vi "server.vi"() -> ()   [LabVIEW 2020]
uses:
  System.Windows.Forms
  TCP Multiple Connections Data.ctl
  <userlib>/_MGI/Menu Building/MenuTypes/MenuStrip/MGI_MenuStrip.lvclass
  <userlib>/_MGI/Menu Building/MenuItemStatusChange/MGI_MenuItemStatusChange.lvclass
panel:
  in  "计划产量":u16 format="%d 件"
  in  "产品型号":u16(ring) items=[""=0, "R128"=1, "R527"=4, "R538"=5, "R92A"=3]
  out "完成率":sgl format="%_3f %"
  out "剩余数量":u16 format="%d 件"
  out "生产数量":u16 format="%d 件"
  out "布尔":bool
  out "停止":bool
  in  "菜单":refnum<k24>(container)
  in  "标题":string="Andon看板"
  out "备份4":T1(xcontrol)
  out "备份3":T1(xcontrol)
  out "备份2":T1(xcontrol)
  out "上转向轴总成、\n上柱管分总成拉拔力检测机":T1(xcontrol)
  out "GP12":T1(xcontrol)
  out "激光检测机":T1(xcontrol)
  out "最终功能测试+NVH 2":T1(xcontrol)
  out "最终功能测试+NVH 1":T1(xcontrol)
  out "传感器检测标定":T1(xcontrol)
  out "调节机构检测":T1(xcontrol)
  out "调节机构螺母拧紧\n扭矩检测机":T1(xcontrol)
  out "上柱管总成装配、\n滑移力检测":T1(xcontrol)
  out "中间轴装配":T1(xcontrol)
  out "控制器支架及电机装配":T1(xcontrol)
  out "上转向轴滑移力检测机":T1(xcontrol)
  out "上转向轴组件压装力检测机":T1(xcontrol)
  out "上/下柱管分总成压装力\n及拧紧扭矩检测机":T1(xcontrol)
  out "上柱管组件压装力检测机":T1(xcontrol)
  out "减速机构NVH测试评价":T1(xcontrol)
  out "双工位磨合试验机":T1(xcontrol)
  out "在线设备":i32 format="%.0d 台"
  # "芜湖恒隆汽车转向系统有限公司"
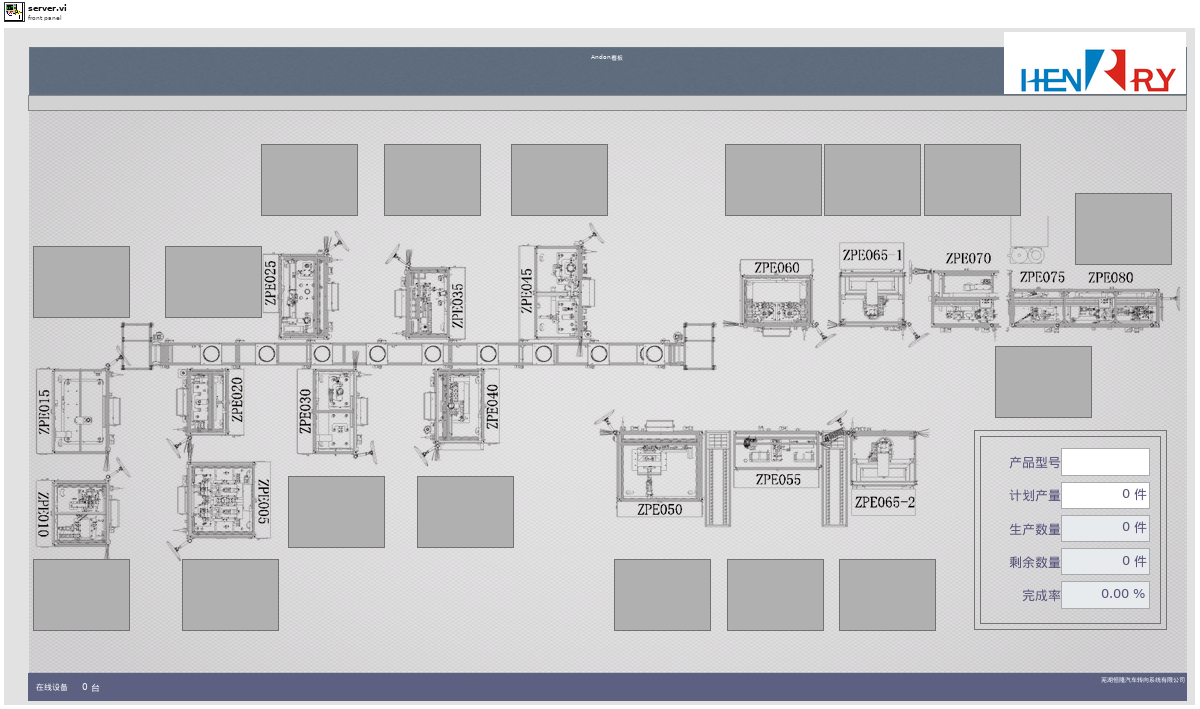
[diagram p1: front panel]
types:
  T1 = cluster{"设备名称":string, "操作人员":string, "设备状态":enum16{"设备离线", "设备正常", "设备缺料", "设备故障", "质量报警"}, "附加信息":string}
  T2 = typedef "TCP Multiple Connections Data.ctl" = cluster{"客户端":refnum<k5>[], "侦听器":refnum<k5>, "上线设备":string[]}
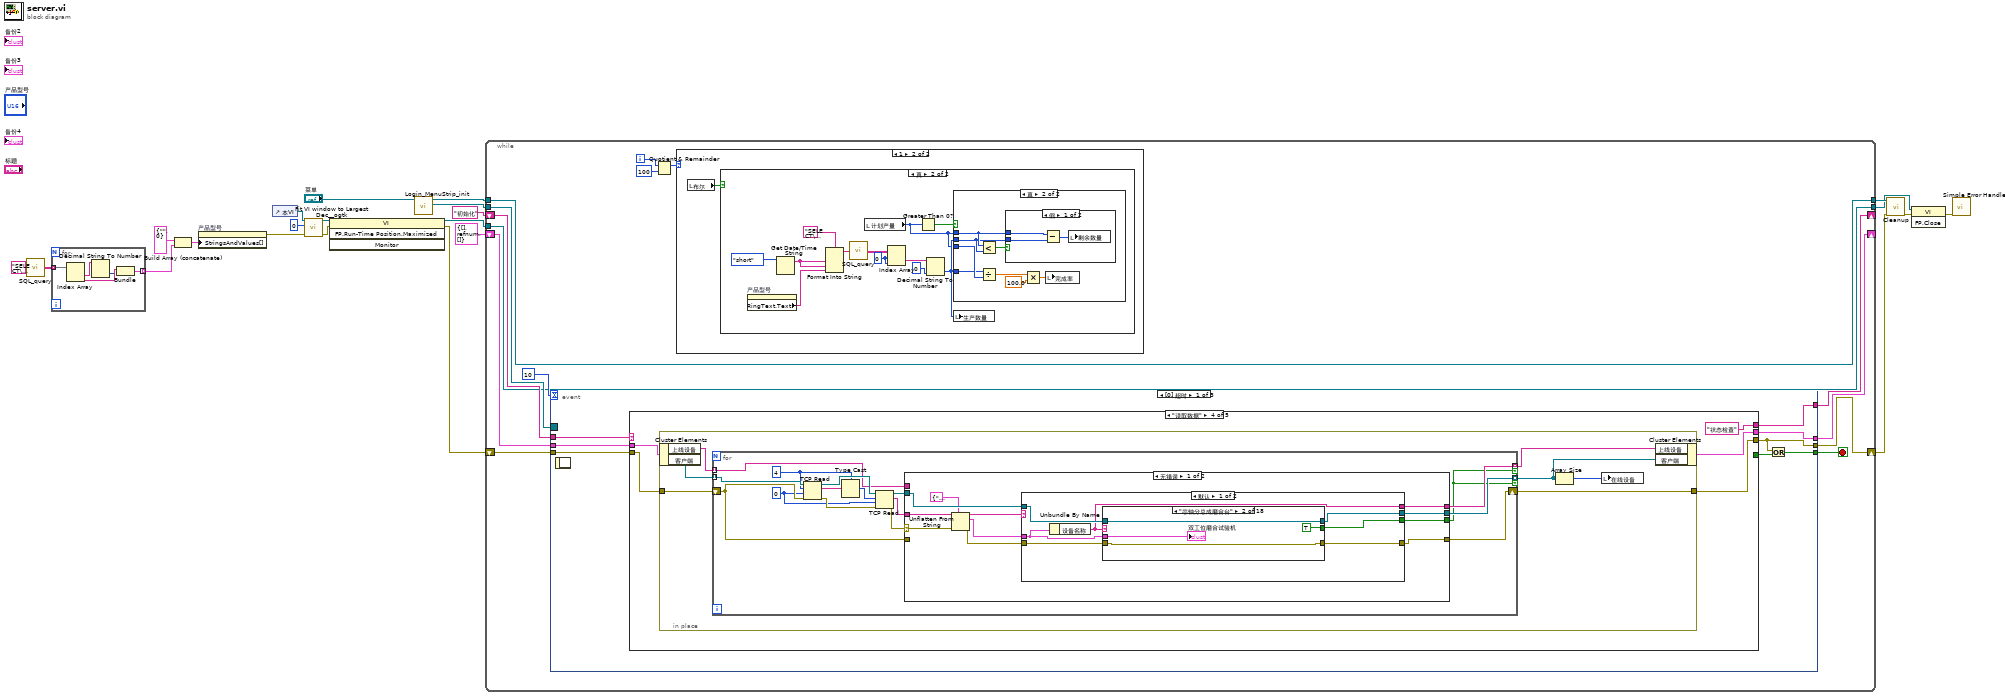
[diagram p0: block diagram]
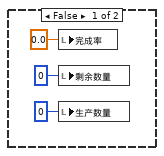
[diagram p3: hidden frame]
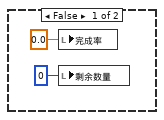
[diagram p4: hidden frame]
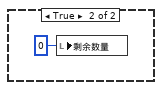
[diagram p5: hidden frame]
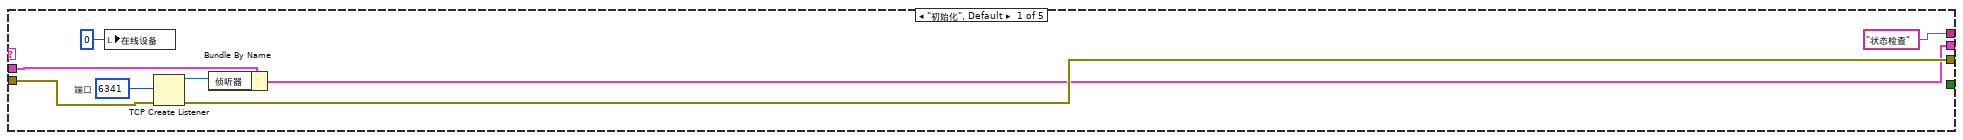
[diagram p6: hidden frame]
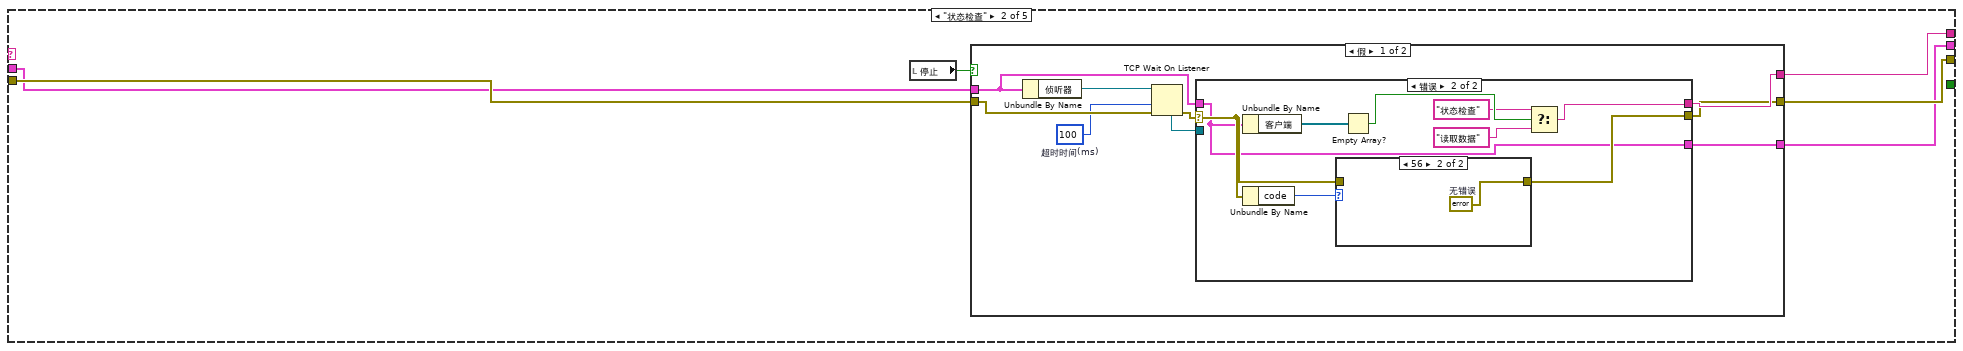
[diagram p7: hidden frame]
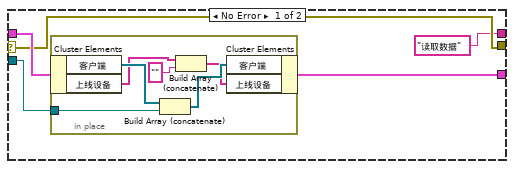
[diagram p8: hidden frame]
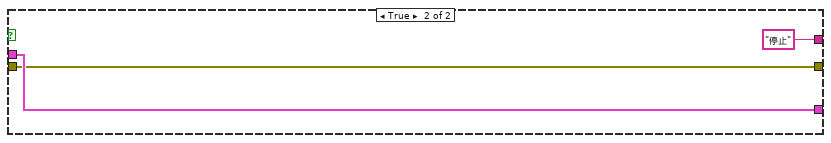
[diagram p10: hidden frame]
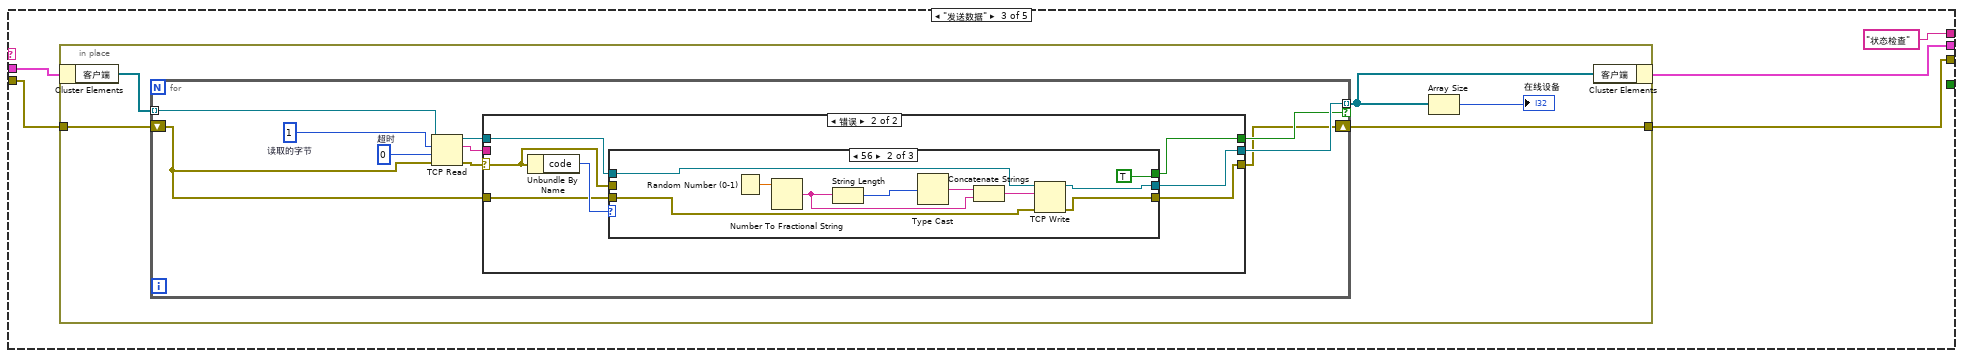
[diagram p11: hidden frame]
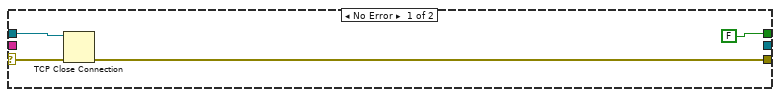
[diagram p12: hidden frame]
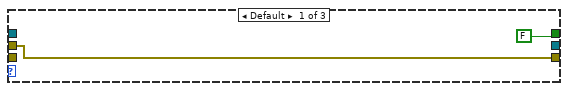
[diagram p13: hidden frame]
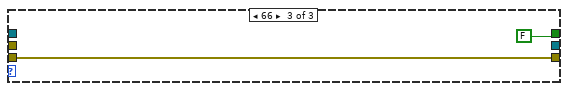
[diagram p14: hidden frame]
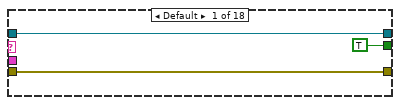
[diagram p15: hidden frame]
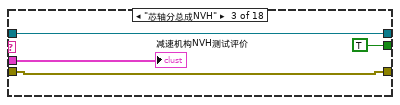
[diagram p16: hidden frame]
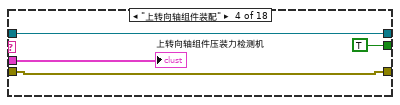
[diagram p17: hidden frame]
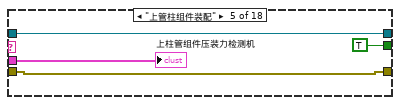
[diagram p18: hidden frame]
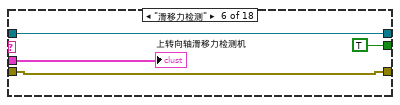
[diagram p19: hidden frame]
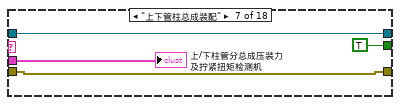
[diagram p20: hidden frame]
diagram:
  n1 = call "SQL_query.vi"("SQL query"="SELECT\ndbo.Product.PRODUCT_ID,\ndbo.Product.PRODUCT_NAME\n\nFROM\ndbo.Product\n") -> ("data"=w3:string[][])  [unwired: 3 in, 1 out]
  n2 = for {
    tunnel: w3 -> [w27] mode=indexing
    tunnel: [w25] -> w6 mode=indexing
    n3 = Index Array(array=w27) -> (element #1=w24:string, element #2=w26:string)  [unwired: 2 in]
    n4 = Decimal String To Number(string=w24) -> (number=w23:i32)  [unwired: 2 in, 1 out]
    n5 = Bundle(w26, w23) -> (w25:cluster{string, i32})  [unwired: 1 in]
  }
  n6 = Build Array (concatenate)(cluster{string, i32} {"", 0}, w6) -> (w2:cluster{string, i32}[])
  n7 = property on="产品型号" class="Ring (严格)"("StringsAndValues[]"=w2) -> (error out=w1:errorcluster)  [unwired: 2 in, 1 out]
  n8 = control-ref of="本VI"() -> (w18:refnum<vi>)
  n9 = call <userlib>:"Fit VI window to Largest Dec__ogtk.vi"("error in (no error)"=w1, "border spacing (2 px)"=0, "VI Ref (calling VI)"=w18) -> ("error out"=w15:errorcluster, "dup VI Ref"=w20:refnum<vi>)  [unwired: 3 in]
  n10 = invoke class="VI" method="FP.Run-Time Position.Maximized"(reference=w20, error in=w15) -> (reference out=w19:refnum<vi>, error out=w14:errorcluster)  [unwired: 2 in, 2 out]
  n11 = call "Login_MenuStrip_init.vi"("MenuStrip"="菜单") -> ("MenuStrip_Event"=w13:refnum<event-registration>, "Menu out"=w12:refnum<class "MGI_MenuStrip.lvclass">)  [unwired: 9 in]
  n12 = while {
    shift-right: [w40] -> _
    shift-left: "初始化" -> [w41]
    shift-right: [w38] -> _
    shift-left: T2 {"客户端"=[], "侦听器"=refnum, "上线设备"=[]} ("数据") -> [w39]
    shift-right: [w35] -> w10
    shift-left: w14 -> [w37]
    tunnel: w19 -> [w31]
    tunnel: w13 -> [w34]
    tunnel: w12 -> [w33]
    tunnel: [w33] -> w11
    tunnel: [w31] -> w9
    i -> [w30]
    stop <- w36 stop-if-true
    n13 = event shown="[0] 超时" {
      selector: w34 -> [_ _ _]
      dyn-events: _ -> [_ _ _]
      timeout: 10 -> [_ _ _]
      tunnel: w41 -> [w79 w382 w389]
      tunnel: [w78 w382 w388] -> w40
      tunnel: w39 -> [w77 w381 w390]
      tunnel: [w76 w381 w390] -> w38
      tunnel: w37 -> [w75 w380 w391]
      tunnel: [w73 _ _] -> w36
      tunnel: [w72 w380 w391] -> w35
      event Timeout {
        n14 = event-data() -> ()  [unwired: 1 in, 1 out]
        n15 = case shown="\"读取数据\"" w79 {
          tunnel: ["状态检查" w93 "状态检查" "状态检查" "停止"] -> w78
          tunnel: [_ _ _ _ TRUE ("停止循环？")] -> w74
          tunnel: w77 -> [w85 w90 w130 w175 w375]
          tunnel: [w84 w89 w129 w174 w375] -> w76
          tunnel: w75 -> [w87 w92 w132 w177 w374]
          tunnel: [w86 w91 w131 w176 w372] -> w72
          frame "初始化", Default {
            w82 = u16 6341  # 端口
            # "创建TCP侦听器函数创建一个侦听器引用，用于检查新客户端连接。"
            n16 = local write "在线设备"(0 ("Number of Client Connections")) -> ()
            n17 = TCP Create Listener(8:w87, 10:w82) -> (0:w86:errorcluster, 3:w83:refnum<k5>)  [unwired: 4 out]
            n18 = Bundle By Name(cluster=w85, "侦听器"=w83) -> (w84:T2)
          }
          frame "状态检查" {
            # "检查“停止”按钮状态，以及连接至该按钮的客户端是否需要数据。"
            n19 = local read "停止"() -> (w88:bool)
            n20 = case shown="假" w88 {
              tunnel: [w102 "停止"] -> w93
              tunnel: w92 -> [w101 w125]
              tunnel: [w100 w125] -> w91
              tunnel: w90 -> [w99 w127]
              tunnel: [w98 w127] -> w89
              frame False {
                w97 = 100  # 超时时间(ms)
                n21 = Unbundle By Name(w99) -> ("侦听器"=w94:refnum<k5>)
                n22 = TCP Wait On Listener(8:w101, 9:w97, 11:w94) -> (0:w96:errorcluster, 4:w95:refnum<k5>)  [unwired: 4 out]
                n23 = case shown="错误" w96 {
                  selector: w96 -> [w105 w122]
                  tunnel: ["读取数据" w116] -> w102
                  tunnel: w95 -> [w106 _]
                  tunnel: w99 -> [w107 w119]
                  tunnel: [w104 w119] -> w98
                  tunnel: [w105 w120] -> w100
                  frame No Error {
                    # "将新客户端连接添加至状态数据并进入'Send Data'状态。"
                    n24 = in-place {
                      in-place-border: w106 -> [w111]
                      n25 = in-place-cluster #1(w107) -> ("客户端"=w113:refnum<k5>[], "上线设备"=w109:string[])
                      n26 = Build Array (concatenate)(w113, w111) -> (w112:refnum<k5>[])
                      n27 = Build Array (concatenate)(w109, "") -> (w108:string[])
                      n28 = in-place-cluster #1("客户端"=w112, "上线设备"=w108) -> (w104:T2)
                    }
                  }
                  frame Error {
                    n29 = Unbundle By Name(w119) -> ("客户端"=w118:refnum<k5>[])
                    n30 = Unbundle By Name(w122) -> ("code"=w121:i32)
                    n31 = case shown="56" w121 {
                      tunnel: w122 -> [w123 _]
                      tunnel: [w123 w124] -> w120
                      frame Default {
                      }
                      frame 56 {
                        w124 = errorcluster {"status"=FALSE, "code"=0, "source"=""}  # 无错误
                      }
                    }
                    n32 = Empty Array?(array=w118) -> (empty?=w117:bool)
                    n33 = Select(t="状态检查", s=w117, f="读取数据") -> (s? t:f=w116:string)
                  }
                }
              }
              frame True {
              }
            }
          }
          frame "发送数据" {
            # "对客户端数组中的每个项执行下列操作：\n(1) 尝试通过读取TCP数据函数从客户端读取一个字节。如发生超时或连接关闭，忽略错误。如客户端返回一个字节，表明已关闭连接。\n(2) 如未发生错误且客户端未返回字节，则使用写入TCP数据函数向客户端发送当前数据。"
            n34 = in-place {
              in-place-border: w132 -> [w137]
              in-place-border: [w136] -> w131
              n35 = in-place-cluster #2(w130) -> ("客户端"=w134:refnum<k5>[])
              n36 = for {
                tunnel: w134 -> [w147] mode=indexing
                shift-right: [w139] -> w136
                shift-left: w137 -> [w138]
                tunnel: [w141] -> w133 mode=indexing if=w140
                w144 = 0  # 超时
                w145 = 1  # 读取的字节
                n37 = TCP Read(connection ID=w147, bytes to read=w145, error in (no error)=w138, 9:w144) -> (connection ID out=w146:refnum<k5>, data out=w142:string, error out=w143:errorcluster)  [unwired: 1 out]
                n38 = case shown="错误" w143 {
                  selector: w143 -> [w150 w157]
                  tunnel: w146 -> [w151 w154]
                  tunnel: w142 -> [_ _]
                  tunnel: [_ w152] -> w141
                  tunnel: [FALSE w153] -> w140
                  tunnel: [w148 w156] -> w139
                  tunnel: w138 -> [_ w155]
                  frame No Error {
                    # "如客户端发送了数据，则通知应关闭连接。"
                    n39 = TCP Close Connection(connection ID=w151, error in (no error)=w150) -> (error out=w148:errorcluster)  [unwired: 2 out]
                  }
                  frame Error {
                    # "忽略连接关闭和超时错误"
                    n40 = Unbundle By Name(w157) -> ("code"=w158:i32)
                    n41 = case shown="56" w158 {
                      tunnel: w157 -> [w160 _ _]
                      tunnel: [w160 w170 w172] -> w156
                      tunnel: w155 -> [_ w166 w172]
                      tunnel: w154 -> [_ w169 _]
                      tunnel: [FALSE TRUE FALSE] -> w153
                      tunnel: [_ w168 _] -> w152
                      frame Default {
                        # "未知错误将直接忽略。"
                      }
                      frame 56 {
                        n42 = Random Number (0-1)() -> (number: 0 to 1=w165:dbl)
                        n43 = Number To Fractional String(number=w165) -> (F-format string=w162:string)  [unwired: 3 in]
                        n44 = String Length(string=w162) -> (length=w163:i32)
                        n45 = Type Cast(x=w163) -> (*(type *) &x=w164:string)  [unwired: 1 in]
                        n46 = Concatenate Strings(w164, w162) -> (w161:string)
                        n47 = TCP Write(connection ID=w169, data in=w161, error in (no error)=w166) -> (connection ID out=w168:refnum<k5>, error out=w170:errorcluster)  [unwired: 2 out]
                      }
                      frame 66 {
                        # "连接关闭，因此该客户端引用句柄不再有效。"
                      }
                    }
                  }
                }
              }
              n48 = Array Size(array=w133) -> (size(s)=→"在线设备":i32)
              n49 = in-place-cluster #2("客户端"=w133) -> (w129:T2)
            }
          }
          frame "读取数据" {
            n50 = in-place {
              in-place-border: w177 -> [w184]
              in-place-border: [w183] -> w176
              n51 = in-place-cluster #3(w175) -> ("上线设备"=w179:string[], "客户端"=w180:refnum<k5>[])
              n52 = for {
                tunnel: w180 -> [w200] mode=indexing
                shift-right: [w198] -> w183
                shift-left: w184 -> [w197]
                tunnel: [w199] -> w181 mode=indexing if=w186
                tunnel: [w187] -> w178 mode=indexing if=w186
                tunnel: w179 -> [w185] mode=indexing
                w189 = 0 ("超时毫秒(25000)")
                w191 = 4 ("读取的字节")
                n53 = TCP Read(connection ID=w200, bytes to read=w191, error in (no error)=w197, 9:w189) -> (connection ID out=w193:refnum<k5>, data out=w192:string, error out=w196:errorcluster)  [unwired: 1 out]
                n54 = Type Cast(type=w191, x=w192) -> (*(type *) &x=w190:i32)
                n55 = TCP Read(connection ID=w193, bytes to read=w190, error in (no error)=w196, 9:w189) -> (connection ID out=w194:refnum<k5>, data out=w188:string, error out=w195:errorcluster)  [unwired: 1 out]
                n56 = case shown="无错误" w195 {
                  selector: w195 -> [w208 w321]
                  tunnel: w194 -> [w211 w318]
                  tunnel: [w202 w316] -> w199
                  tunnel: [w210 w317] -> w186
                  tunnel: [w209 w320] -> w198
                  tunnel: w197 -> [_ w319]
                  tunnel: w188 -> [w207 _]
                  tunnel: [w201 w314] -> w187
                  tunnel: w185 -> [_ w315]
                  frame No Error {
                    # "如客户端发送了数据，则通知应关闭连接。"
                    n57 = Unflatten From String(type=T1 {"设备名称"="", "操作人员"="", "设备状态"=enum."设备离线", "附加信息"=""} ("设备信息"), binary string=w207, error in (no error)=w208) -> (rest of the binary string=w204:string, value=w203:T1, error out=w205:errorcluster)  [unwired: 2 in]
                    n58 = case shown="默认" w204 {
                      tunnel: w211 -> [w215 w296]
                      tunnel: [w218 FALSE] -> w210
                      tunnel: [w214 w294] -> w209
                      tunnel: w205 -> [w213 w293]
                      tunnel: w203 -> [w217 w291]
                      tunnel: [w216 _] -> w202
                      tunnel: [w212 _] -> w201
                      frame Default {
                        n59 = Unbundle By Name(w217) -> ("设备名称"=w212:string)
                        n60 = case shown="\"芯轴分总成磨合台\"" w212 {
                          tunnel: [TRUE TRUE TRUE TRUE TRUE TRUE TRUE TRUE TRUE TRUE TRUE TRUE TRUE TRUE TRUE TRUE TRUE TRUE] -> w218
                          tunnel: w217 -> [_ w222 w226 w230 w234 w238 w242 w246 w250 w254 w258 w262 w266 w270 w274 w278 w282 w286]
                          tunnel: [w221 w224 w228 w232 w236 w240 w244 w248 w252 w256 w260 w264 w268 w272 w276 w280 w284 w289] -> w216
                          tunnel: w215 -> [w221 w224 w228 w232 w236 w240 w244 w248 w252 w256 w260 w264 w268 w272 w276 w280 w284 w289]
                          tunnel: [w220 w223 w227 w231 w235 w239 w243 w247 w251 w255 w259 w263 w267 w271 w275 w279 w283 w288] -> w214
                          tunnel: w213 -> [w220 w223 w227 w231 w235 w239 w243 w247 w251 w255 w259 w263 w267 w271 w275 w279 w283 w288]
                          frame Default {
                          }
                          frame "芯轴分总成磨合台" {
                            "双工位磨合试验机" <- w222
                          }
                          frame "芯轴分总成NVH" {
                            "减速机构NVH测试评价" <- w226
                          }
                          frame "上转向轴组件装配" {
                            "上转向轴组件压装力检测机" <- w230
                          }
                          frame "上管柱组件装配" {
                            "上柱管组件压装力检测机" <- w234
                          }
                          frame "滑移力检测" {
                            "上转向轴滑移力检测机" <- w238
                          }
                          frame "上下管柱总成装配" {
                            "上/下柱管分总成压装力\n及拧紧扭矩检测机" <- w242
                          }
                          frame "滑移力复检" {
                            "上柱管总成装配、\n滑移力检测" <- w246
                          }
                          frame "调节机构装配" {
                            "调节机构螺母拧紧\n扭矩检测机" <- w250
                          }
                          frame "调节机构检测" {
                            "调节机构检测" <- w254
                          }
                          frame "传感器对中台" {
                            "传感器检测标定" <- w258
                          }
                          frame "电机ECU装配" {
                            "控制器支架及电机装配" <- w262
                          }
                          frame "最终性能试验台1" {
                            "最终功能测试+NVH 1" <- w266
                          }
                          frame "最终性能试验台2" {
                            "最终功能测试+NVH 2" <- w270
                          }
                          frame "激光打标" {
                            "激光检测机" <- w274
                          }
                          frame "GP12终检" {
                            "GP12" <- w278
                          }
                          frame "中间轴装配" {
                            "中间轴装配" <- w282
                          }
                          frame "上管柱上转向轴合成" {
                            "上转向轴总成、\n上柱管分总成拉拔力检测机" <- w286
                          }
                        }
                      }
                      frame "Q" {
                        n61 = Unbundle By Name(w291) -> ("设备名称"=w290:string)
                        n62 = TCP Close Connection(connection ID=w296, error in (no error)=w293) -> (error out=w294:errorcluster)  [unwired: 2 out]
                        n63 = case shown="\"上转向轴组件装配\"" w290 {
                          tunnel: T1 {"设备名称"="", "操作人员"="", "设备状态"=enum."设备离线", "附加信息"=""} ("芯轴分总成磨合台") -> [_ w297 w298 w299 w300 w301 w302 w303 w304 w305 w306 w307 w308 w309 w310 w311 w312 w313]
                          frame Default {
                          }
                          frame "芯轴分总成磨合台" {
                            n64 = local write "双工位磨合试验机"(w297) -> ()
                          }
                          frame "芯轴分总成NVH" {
                            n65 = local write "减速机构NVH测试评价"(w298) -> ()
                          }
                          frame "上转向轴组件装配" {
                            n66 = local write "上转向轴组件压装力检测机"(w299) -> ()
                          }
                          frame "上管柱组件装配" {
                            n67 = local write "上柱管组件压装力检测机"(w300) -> ()
                          }
                          frame "滑移力检测" {
                            n68 = local write "上转向轴滑移力检测机"(w301) -> ()
                          }
                          frame "上下管柱总成装配" {
                            n69 = local write "上/下柱管分总成压装力\n及拧紧扭矩检测机"(w302) -> ()
                          }
                          frame "滑移力复检" {
                            n70 = local write "上柱管总成装配、\n滑移力检测"(w303) -> ()
                          }
                          frame "调节机构装配" {
                            n71 = local write "调节机构螺母拧紧\n扭矩检测机"(w304) -> ()
                          }
                          frame "调节机构检测" {
                            n72 = local write "调节机构检测"(w305) -> ()
                          }
                          frame "传感器对中台" {
                            n73 = local write "传感器检测标定"(w306) -> ()
                          }
                          frame "电机ECU装配" {
                            n74 = local write "控制器支架及电机装配"(w307) -> ()
                          }
                          frame "最终性能试验台1" {
                            n75 = local write "最终功能测试+NVH 1"(w308) -> ()
                          }
                          frame "最终性能试验台2" {
                            n76 = local write "最终功能测试+NVH 2"(w309) -> ()
                          }
                          frame "激光打标" {
                            n77 = local write "激光检测机"(w310) -> ()
                          }
                          frame "GP12终检" {
                            n78 = local write "GP12"(w311) -> ()
                          }
                          frame "中间轴装配" {
                            n79 = local write "中间轴装配"(w312) -> ()
                          }
                          frame "上管柱上转向轴合成" {
                            n80 = local write "上转向轴总成、\n上柱管分总成拉拔力检测机"(w313) -> ()
                          }
                        }
                      }
                    }
                  }
                  frame Error {
                    # "忽略连接关闭和超时错误"
                    n81 = Unbundle By Name(w321) -> ("code"=w322:i32)
                    n82 = case shown="66" w322 {
                      tunnel: w321 -> [_ _ _]
                      tunnel: [w323 w346 w351] -> w320
                      tunnel: w319 -> [w323 w346 w351]
                      tunnel: w318 -> [_ w347 _]
                      tunnel: [FALSE TRUE FALSE] -> w317
                      tunnel: [_ w347 _] -> w316
                      tunnel: w315 -> [w324 w344 w348]
                      tunnel: [_ w344 _] -> w314
                      frame Default {
                        # "未知错误将直接忽略。"
                        n83 = case shown="\"上转向轴组件装配\"" w324 {
                          tunnel: T1 {"设备名称"="", "操作人员"="", "设备状态"=enum."设备离线", "附加信息"=""} ("芯轴分总成磨合台") -> [_ w327 w328 w329 w330 w331 w332 w333 w334 w335 w336 w337 w338 w339 w340 w341 w342 w343]
                          frame Default {
                          }
                          frame "芯轴分总成磨合台" {
                            n84 = local write "双工位磨合试验机"(w327) -> ()
                          }
                          frame "芯轴分总成NVH" {
                            n85 = local write "减速机构NVH测试评价"(w328) -> ()
                          }
                          frame "上转向轴组件装配" {
                            n86 = local write "上转向轴组件压装力检测机"(w329) -> ()
                          }
                          frame "上管柱组件装配" {
                            n87 = local write "上柱管组件压装力检测机"(w330) -> ()
                          }
                          frame "滑移力检测" {
                            n88 = local write "上转向轴滑移力检测机"(w331) -> ()
                          }
                          frame "上下管柱总成装配" {
                            n89 = local write "上/下柱管分总成压装力\n及拧紧扭矩检测机"(w332) -> ()
                          }
                          frame "滑移力复检" {
                            n90 = local write "上柱管总成装配、\n滑移力检测"(w333) -> ()
                          }
                          frame "调节机构装配" {
                            n91 = local write "调节机构螺母拧紧\n扭矩检测机"(w334) -> ()
                          }
                          frame "调节机构检测" {
                            n92 = local write "调节机构检测"(w335) -> ()
                          }
                          frame "传感器对中台" {
                            n93 = local write "传感器检测标定"(w336) -> ()
                          }
                          frame "电机ECU装配" {
                            n94 = local write "控制器支架及电机装配"(w337) -> ()
                          }
                          frame "最终性能试验台1" {
                            n95 = local write "最终功能测试+NVH 1"(w338) -> ()
                          }
                          frame "最终性能试验台2" {
                            n96 = local write "最终功能测试+NVH 2"(w339) -> ()
                          }
                          frame "激光打标" {
                            n97 = local write "激光检测机"(w340) -> ()
                          }
                          frame "GP12终检" {
                            n98 = local write "GP12"(w341) -> ()
                          }
                          frame "中间轴装配" {
                            n99 = local write "中间轴装配"(w342) -> ()
                          }
                          frame "上管柱上转向轴合成" {
                            n100 = local write "上转向轴总成、\n上柱管分总成拉拔力检测机"(w343) -> ()
                          }
                        }
                      }
                      frame 56 {
                      }
                      frame 66 {
                        # "连接关闭，因此该客户端引用句柄不再有效。"
                        n101 = case shown="\"上转向轴组件装配\"" w348 {
                          tunnel: T1 {"设备名称"="", "操作人员"="", "设备状态"=enum."设备离线", "附加信息"=""} ("芯轴分总成磨合台") -> [_ w352 w353 w354 w355 w356 w357 w358 w359 w360 w361 w362 w363 w364 w365 w366 w367 w368]
                          frame Default {
                          }
                          frame "芯轴分总成磨合台" {
                            n102 = local write "双工位磨合试验机"(w352) -> ()
                          }
                          frame "芯轴分总成NVH" {
                            n103 = local write "减速机构NVH测试评价"(w353) -> ()
                          }
                          frame "上转向轴组件装配" {
                            n104 = local write "上转向轴组件压装力检测机"(w354) -> ()
                          }
                          frame "上管柱组件装配" {
                            n105 = local write "上柱管组件压装力检测机"(w355) -> ()
                          }
                          frame "滑移力检测" {
                            n106 = local write "上转向轴滑移力检测机"(w356) -> ()
                          }
                          frame "上下管柱总成装配" {
                            n107 = local write "上/下柱管分总成压装力\n及拧紧扭矩检测机"(w357) -> ()
                          }
                          frame "滑移力复检" {
                            n108 = local write "上柱管总成装配、\n滑移力检测"(w358) -> ()
                          }
                          frame "调节机构装配" {
                            n109 = local write "调节机构螺母拧紧\n扭矩检测机"(w359) -> ()
                          }
                          frame "调节机构检测" {
                            n110 = local write "调节机构检测"(w360) -> ()
                          }
                          frame "传感器对中台" {
                            n111 = local write "传感器检测标定"(w361) -> ()
                          }
                          frame "电机ECU装配" {
                            n112 = local write "控制器支架及电机装配"(w362) -> ()
                          }
                          frame "最终性能试验台1" {
                            n113 = local write "最终功能测试+NVH 1"(w363) -> ()
                          }
                          frame "最终性能试验台2" {
                            n114 = local write "最终功能测试+NVH 2"(w364) -> ()
                          }
                          frame "激光打标" {
                            n115 = local write "激光检测机"(w365) -> ()
                          }
                          frame "GP12终检" {
                            n116 = local write "GP12"(w366) -> ()
                          }
                          frame "中间轴装配" {
                            n117 = local write "中间轴装配"(w367) -> ()
                          }
                          frame "上管柱上转向轴合成" {
                            n118 = local write "上转向轴总成、\n上柱管分总成拉拔力检测机"(w368) -> ()
                          }
                        }
                      }
                    }
                  }
                }
              }
              n119 = Array Size(array=w181) -> (size(s)=w182:i32)
              n120 = local write "在线设备"(w182) -> ()
              n121 = in-place-cluster #3("上线设备"=w178, "客户端"=w181) -> (w174:T2)
            }
          }
          frame "停止" {
            # "通过关闭TCP连接函数关闭所有打开的客户端和侦听器连接。"
            n122 = Unbundle By Name(w375) -> ("客户端"=w373:refnum<k5>[], "侦听器"=w370:refnum<k5>)
            n123 = TCP Close Connection(connection ID=w370, error in (no error)=w374) -> (error out=w371:errorcluster)  [unwired: 1 in, 1 out]
            n124 = for {
              shift-right: [w378] -> w372
              shift-left: w371 -> [w379]
              tunnel: w373 -> [w377] mode=indexing
              n125 = TCP Close Connection(connection ID=w377, error in (no error)=w379) -> (error out=w378:errorcluster)  [unwired: 1 in, 1 out]
            }
            n126 = Quit LabVIEW() -> ()  [unwired: 1 in]
          }
        }
        n127 = Or(x=w72, y=w74) -> (x .or. y?=w73:bool)
      }
      event "产品型号": Value Change {
        n128 = event-data() -> ("NewVal"=w384:u16)  [unwired: 1 in, 5 out]
        n129 = case shown="默认" w384 {
          tunnel: [FALSE TRUE] -> w383
          frame 0 {
          }
          frame Default {
          }
        }
        "布尔" <- w383
      }
      event User Event {
        n130 = event-data() -> ("StatusChange"=w393:refnum<class "MGI_MenuItemStatusChange.lvclass">)  [unwired: 1 in]
        n131 = call <userlib>:"BasicInfo.vi"("MGI_MenuItemStatusChange in"=w393) -> ("Tag"=w392:string)  [unwired: 7 in, 3 out]
        n132 = case shown="\"退出\"" w392 {
          tunnel: w389 -> [w394 _]
          tunnel: [w394 "停止"] -> w388
          tunnel: [_ TRUE ("停止")] -> w387
          frame Default {
          }
          frame "退出" {
            n133 = Quit LabVIEW() -> ()  [unwired: 1 in]
          }
        }
        "停止" <- w387
      }
    }
    n134 = Quotient & Remainder(x=w30, y=100) -> (x-y*floor(x/y)=w28:i32)  [unwired: 1 out]
    n135 = case shown="1" w28 {
      frame 0, Default {
      }
      frame 1 {
        n136 = local read "布尔"() -> (w42:bool)
        n137 = case shown="真" w42 {
          frame False {
            n138 = local write "完成率"(sgl 0.0 ("完成率")) -> ()
            n139 = local write "剩余数量"(u16 0 ("剩余数量")) -> ()
            n140 = local write "生产数量"(u16 0 ("生产数量")) -> ()
          }
          frame True {
            w51 = 0 ("索引 (行)")
            n141 = property on="产品型号" class="Ring (严格)"() -> ("RingText.Text"=w54:string)  [unwired: 2 in, 2 out]
            n142 = Get Date/Time String(date format (0)=enum16{"short", "long", "abbreviated"}."short" ("日期格式(0)")) -> (date string=w53:string)  [unwired: 2 in, 1 out]
            n143 = Format Into String(format string="SELECT\ncount(*)\n\nFROM\ndbo.Result\nINNER JOIN dbo.Code ON dbo.Result.CODE_ID = dbo.Code.CODE_ID\nINNER JOIN dbo.Product ON dbo.Code.PRODUCT_ID = dbo.Product.PRODUCT_ID\nWHERE\ndbo.Result.DEVICE_ID = 22 AND\ndbo.Result.RESULT_TIME BETWEEN '%s 00:00:00' AND '%s 23:59:59' AND\ndbo.Product.PRODUCT_NAME = '%s'" ("格式字符串"), w53, w53, w54) -> (resulting string=w52:string)  [unwired: 2 in, 1 out]
            n144 = call "SQL_query.vi"("SQL query"=w52) -> ("data"=w55:string[][])  [unwired: 3 in, 1 out]
            n145 = local read "计划产量"() -> (w46:u16)
            n146 = Index Array(array=w55, index (row)=w51, index (col)=w51) -> (element=w56:string)
            n147 = Greater Than 0?(x=w46) -> (x > 0?=w57:bool)
            n148 = Decimal String To Number(string=w56, default (0L)=u16 0 ("默认(0 I32)")) -> (number=w47:u16)  [unwired: 1 in, 1 out]
            n149 = case shown="真" w57 {
              tunnel: w46 -> [_ w65]
              tunnel: w47 -> [_ w64]
              tunnel: w47 -> [_ w61]
              tunnel: w46 -> [_ w62]
              frame False {
                n150 = local write "完成率"(sgl 0.0 ("完成率")) -> ()
                n151 = local write "剩余数量"(u16 0 ("剩余数量")) -> ()
              }
              frame True {
                n152 = Less?(x=w62, y=w61) -> (x < y?=w60:bool)
                n153 = Divide(x=w64, y=w65) -> (x/y=w63:dbl)
                n154 = case shown="假" w60 {
                  tunnel: w61 -> [w70 _]
                  tunnel: w62 -> [w69 _]
                  frame False {
                    n155 = Subtract(x=w69, y=w70) -> (x-y=w68:u16)
                    n156 = local write "剩余数量"(w68) -> ()
                  }
                  frame True {
                    n157 = local write "剩余数量"(i16 0 ("剩余数量")) -> ()
                  }
                }
                n158 = Multiply(x=w63, y=100.0) -> (x*y=w66:dbl)
                n159 = local write "完成率"(w66) -> ()
              }
            }
            n160 = local write "生产数量"(w47) -> ()
          }
        }
      }
    }
  }
  n161 = call-dynamic "Cleanup.vi"("error in (no error)"=w10, "MenuStrip in"=w11) -> ("error out"=w8:errorcluster)  [unwired: 9 in]
  n162 = invoke class="VI" method="FP.Close"(reference=w9, error in=w8) -> (error out=w7:errorcluster)  [unwired: 1 in, 2 out]
  n163 = call <vilib>:"Simple Error Handler.vi"("error in (no error)"=w7) -> ()  [unwired: 4 in, 5 out]
